vi "EMD8216 security status read.vi"(11 "CardID":u32) -> (2 "lock_status":u8, 3 "error_code":u32)   [LabVIEW 2009, in "EMD8216_64.lvlib"]
doc: "EMD8216Status EMD8216_security_status_read(u32 CardID,u8 *lock_status);"
uses:
  EMD8216_64.lvlib
  <userlib>/EMD8216_64/EMD8216_64.dll
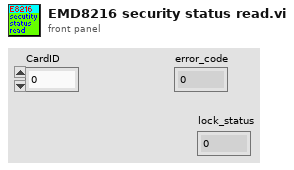
[diagram p1: front panel]
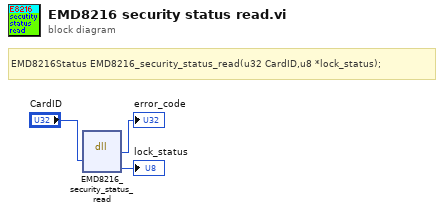
[diagram p0: block diagram]
diagram:
  # "EMD8216Status EMD8216_security_status_read(u32 CardID,u8 *lock_status);"
  n1 = dll-call lib="C:/Program Files/National Instruments/LabVIEW 2017/user.lib/EMD8216_64/EMD8216_64.*" fn="EMD8216_security_status_read"("CardID"="CardID") -> ("return type"=→"error_code":u32, "lock_status"=→"lock_status":u8)  [unwired: 5 in, 2 out]
